vi "GetChannelsMMS.vi"(8 "error in (no error)":errorcluster) -> (0 "error out":errorcluster, 1 "found":bool, 2 "non-shared data groups":string[](array[string]), 3 "MMS Channels":T1[](array[typedef]), 4 "shared data group exists?":bool)   [LabVIEW 2017, in "McsaVirtualChannel.lvlib"]
uses:
  <vilib>/addons/InsightCM/Devices/Shared/Mcsa/McsaVirtualChannel/McsaVirtualChannel.lvlib
  <vilib>/addons/InsightCM/MessageBus/Base/controls/R2_Channel.ctl
  <vilib>/addons/InsightCM/MessageBus/Base/controls/KeyValuePair.ctl
  <vilib>/addons/InsightCM/MessageBus/Base/controls/Metric.ctl
  <vilib>/addons/InsightCM/Utilities/GlobalConfiguration/GlobalConfiguration.lvlib
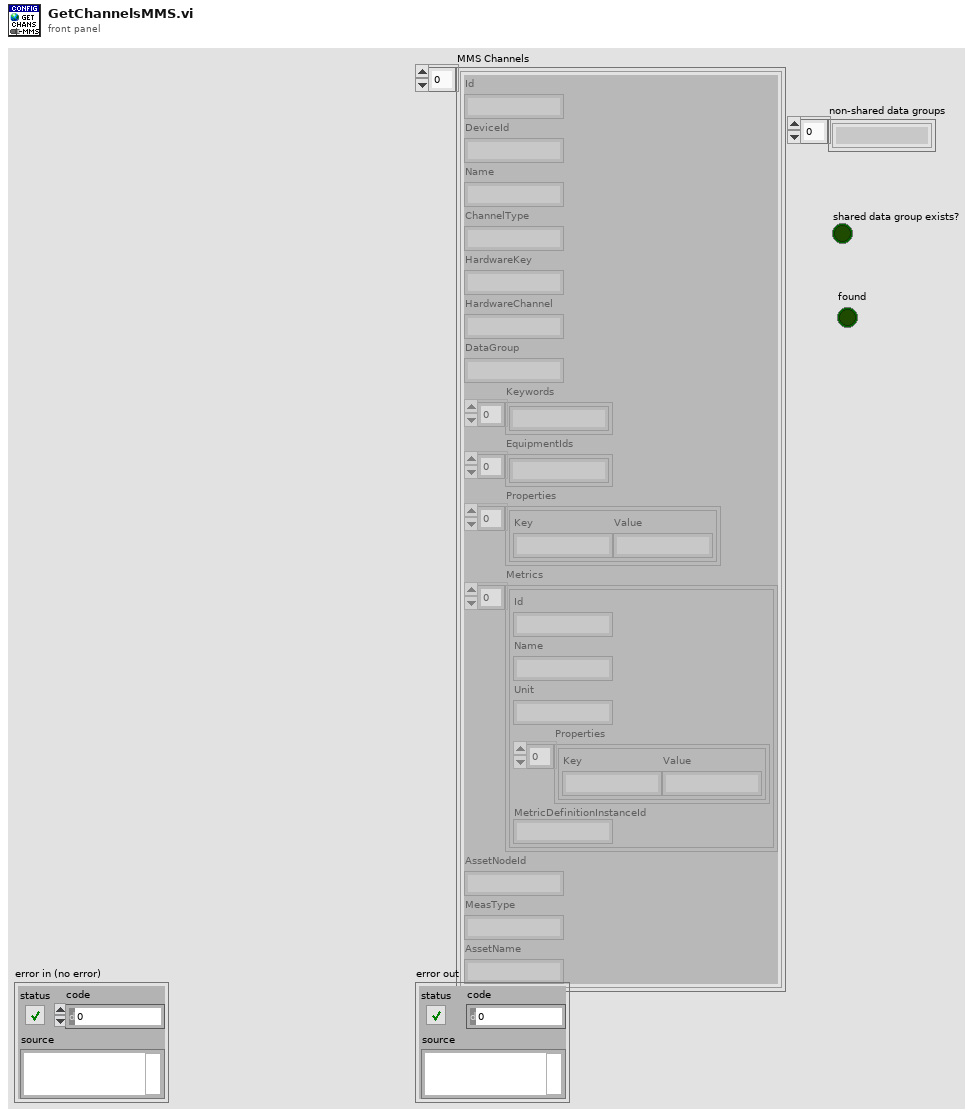
[diagram p1: front panel]
types:
  T1 = typedef "R2_Channel.ctl" = cluster{"Id":string, "DeviceId":string, "Name":string, "ChannelType":string, "HardwareKey":string, "HardwareChannel":string, "DataGroup":string, "Keywords":string[], "EquipmentIds":string[], "Properties":T2[], "Metrics":T3[], "AssetNodeId":string, "MeasType":string, "AssetName":string}
  T2 = typedef "KeyValuePair.ctl" = cluster{"Key":string, "Value":string}
  T3 = typedef "Metric.ctl" = cluster{"Id":string, "Name":string, "Unit":string, "Properties":T2[], "MetricDefinitionInstanceId":string}
  T4 = typedef "AssetNode.ctl" = cluster{"Id":string, "Type":string, "Name":string, "ParentIds":string[], "State":T5, "MeasType":string, "Properties":T2[], "OperatingStates":T6[], "Metrics":T3[], "TrendAlarmRules":T9[], "References":T12[]}
  T5 = typedef "AssetState.ctl" = cluster{"Disabled":bool}
  T6 = typedef "OperatingState.ctl" = cluster{"Name":string, "Properties":T2[], "Triggers":T7[]}
  T7 = typedef "Trigger.ctl" = cluster{"Type":string, "Expression":string, "Conditions":T8[]}
  T8 = typedef "Condition.ctl" = cluster{"Source":string, "Type":string, "Operator":string, "CompareTo":string, "DwellSeconds":dbl}
  T9 = typedef "TrendAlarmRule.ctl" = cluster{"Id":string, "AssetNodeId":string, "TrendId":string, "Disabled":bool, "OperatingState":string, "Operator":string, "Hysteresis":dbl, "OnDelaySeconds":dbl, "OffDelaySeconds":dbl, "Levels":T10[], "Properties":T2[]}
  T10 = typedef "TrendAlarmLevel.ctl" = cluster{"Severity":i32, "CompareTo":dbl, "Actions":T11[]}
  T11 = typedef "AlarmAction.ctl" = cluster{"Type":string, "Props":T2[]}
  T12 = typedef "AssetNodeReference.ctl" = cluster{"NodeId":string, "Name":string}
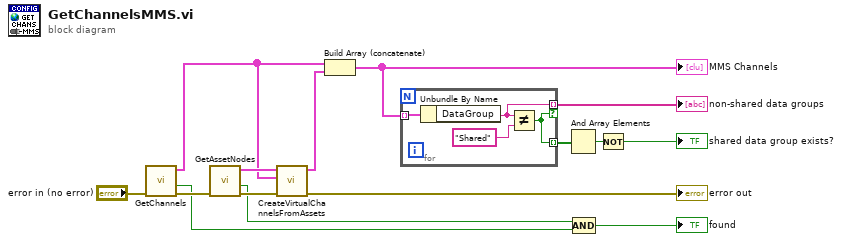
[diagram p0: block diagram]
diagram:
  n1 = call <vilib>:"GetChannels.vi"("error in (no error)"="error in (no error)") -> ("error out"=w10:errorcluster, "found"=w7:bool, "channels"=w9:T1[])  [unwired: 8 in]
  n2 = call <vilib>:"GetAssetNodes.vi"("error in (no error)"=w10) -> ("error out"=w14:errorcluster, "found"=w8:bool, "AssetNodes"=w12:T4[])  [unwired: 8 in]
  n3 = call <vilib>:"CreateVirtualChannelsFromAssets.vi"("error in (no error)"=w14, "Channels"=w9, "AssetNodes"=w12) -> ("error out"=→"error out":errorcluster, "new virtual channels"=w13:T1[])  [unwired: 7 in]
  n4 = Build Array (concatenate)(w9, w13) -> (w5:T1[])
  "MMS Channels" <- w5
  n5 = for {
    tunnel: w5 -> [w19] mode=indexing
    tunnel: [w17] -> w4 mode=indexing if=w16
    tunnel: [w16] -> w3 mode=indexing
    n6 = Unbundle By Name(w19) -> ("DataGroup"=w17:string)
    n7 = Not Equal?(x=w17, y="Shared") -> (x != y?=w16:bool)
  }
  "non-shared data groups" <- w4
  n8 = And Array Elements(Boolean array=w3) -> (logical AND=w2:bool)
  n9 = Compound Arithmetic op=AND(w8, w7) -> (→"found":bool)
  n10 = Not(x=w2) -> (.not. x?=→"shared data group exists?":bool)
